vi "Write Teller.vi"(10 "Teller":refnum<class "Teller.lvclass">, 11 "Stop Msg in":refnum<class "Stop Msg.lvclass">) -> (3 "Stop Msg out":refnum<class "Stop Msg.lvclass">)   [LabVIEW 2025, in "jettl.lvlib" / "Stop jettl Msg.lvlib" / "Stop Msg.lvlib" / "Stop Msg.lvclass"]
uses:
  Stop Msg.lvclass
  Teller/Teller.lvclass
  Stop Msg.lvclass/Stop Msg.ctl
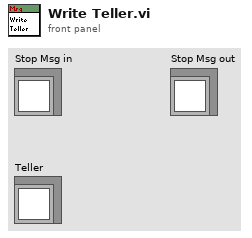
[diagram p1: front panel]
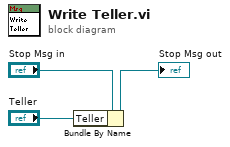
[diagram p0: block diagram]
diagram:
  n1 = Bundle By Name(cluster="Stop Msg in", "Teller"="Teller") -> (→"Stop Msg out":refnum<class "Stop Msg.lvclass">)
